vi "Untitled 1.vi"() -> ()   [LabVIEW 2024]
panel:
  in  "OK Button":bool
  out "Number of Rows":u32
  out "Item Symbols":i32[](array[numeric])
  in  "tbTestData":i32(listbox)
  out "TestDataCurve":T1(graph)
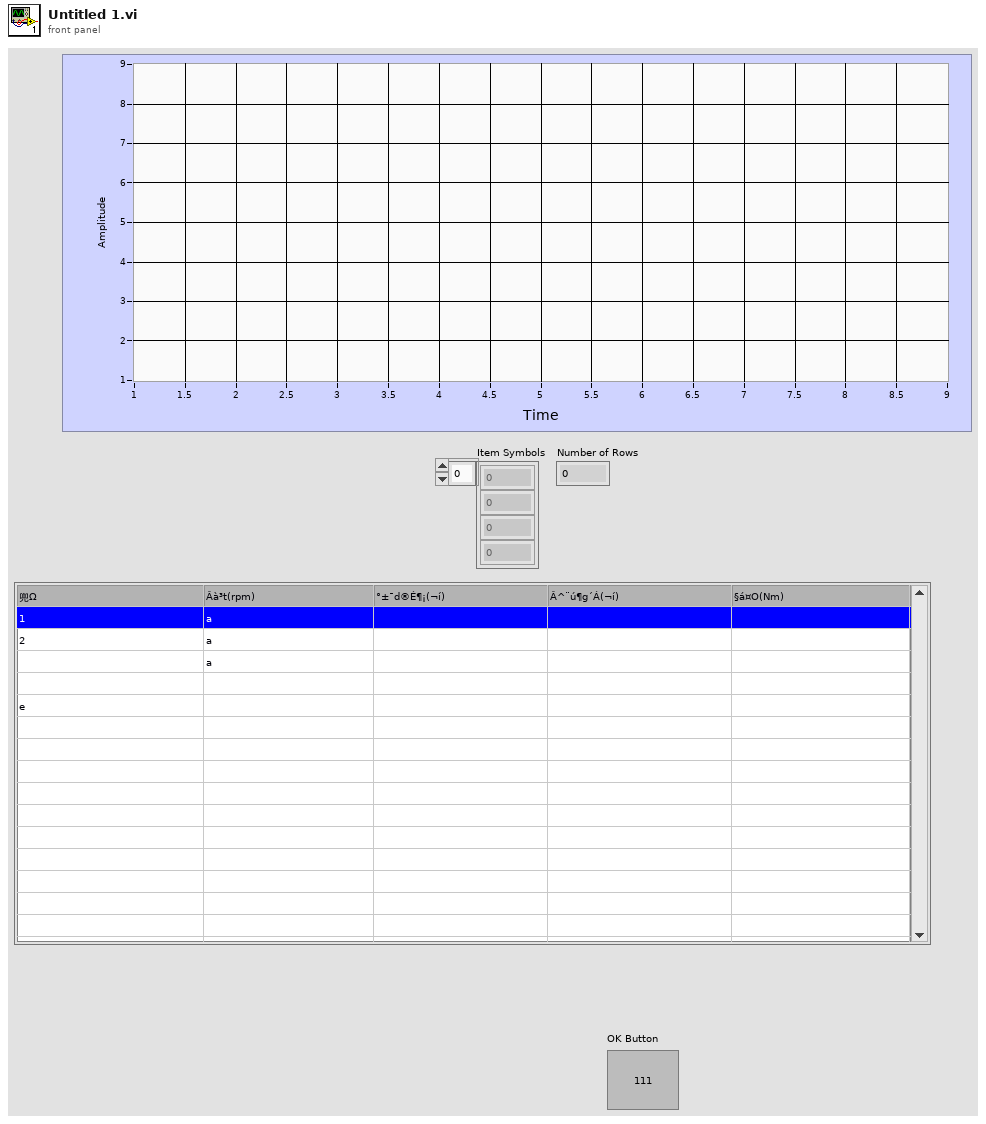
[diagram p1: front panel]
types:
  T1 = cluster{"GraphTestData":dbl[], "GraphTestData":dbl[]}[]
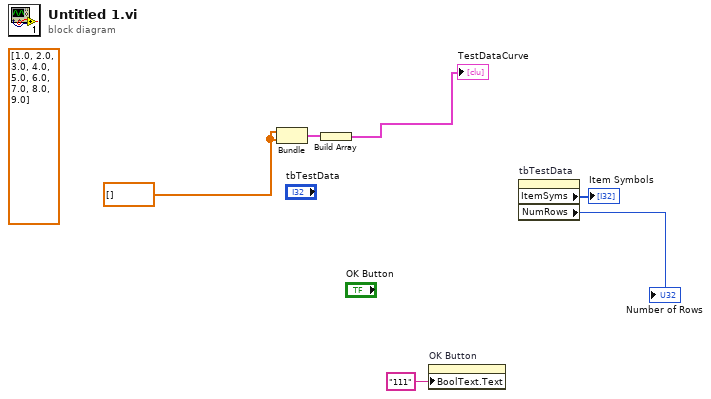
[diagram p0: block diagram]
diagram:
  w2 = dbl[] []
  (unwired) dbl[] [1.0, 2.0, 3.0, 4.0, 5.0, 6.0, 7.0, 8.0, 9.0] ("GraphTestData")
  n1 = Bundle(w2, w2) -> (w6:cluster{dbl[], dbl[]})  [unwired: 1 in]
  n2 = Build Array(w6) -> (→"TestDataCurve":cluster{dbl[], dbl[]}[])
  n3 = property on="OK Button" class="Bool"("BoolText.Text"="111" ("Boolean Text.Text")) -> ()  [unwired: 2 in, 2 out]
  n4 = property on="tbTestData" class="MCListbox (strict)"() -> ("ItemSyms"=→"Item Symbols":i32[], "NumRows"=→"Number of Rows":u32)  [unwired: 2 in, 2 out]
